vi "Check Local uService Status.vi"(8 "error in (no error)":errorcluster, 10 "uService ID":string, 11 "Father of all uServices in":refnum<class "Father of all uServices.lvclass">) -> (0 "error out":errorcluster, 1 "Last Pat":timestamp, 2 "Online?":bool, 3 "Father of all uServices out":refnum<class "Father of all uServices.lvclass">)   [LabVIEW 2020, in "TALOS.lvlib" / "Father of all uServices.lvlib" / "Father of all uServices.lvclass"]
doc: "This VI check the status of a uService, returning Online? if correctly running, and when it was last checked."
uses:
  Father of all uServices.lvclass
  Ancestor/Ancestor/Ancestor.lvclass
  Father of all uServices.lvclass/Father of all uServices.ctl
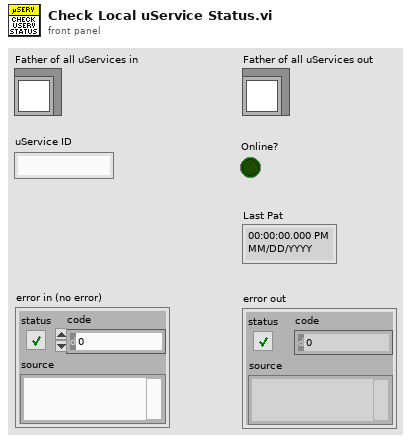
[diagram p1: front panel]
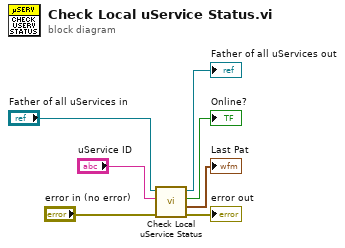
[diagram p0: block diagram]
diagram:
  n1 = call-parent "Check Local uService Status.vi"("error in (no error)"="error in (no error)", "uService ID"="uService ID", "Ancestor in"="Father of all uServices in") -> ("error out"=→"error out":errorcluster, "Last Pat"=→"Last Pat":timestamp, "Online?"=→"Online?":bool, "Ancestor out"=→"Father of all uServices out":refnum<class "Father of all uServices.lvclass">)  [unwired: 5 in]
